vi "Sample Push go for State.vi"(4 "Publish? (T)":bool=TRUE, 6 "Really? (T)":bool=TRUE, 8 "error in (no error)":errorcluster, 9 "State Timeout (Inf=no timeout )":dbl=inf, 10 "Sample Push State":T1=enum."Idle", 11 "cRIO-CO2 in":refnum<class "cRIO-CO2.lvclass">) -> (0 "error out":errorcluster, 3 "cRIO-CO2 out":refnum<class "cRIO-CO2.lvclass">)   [LabVIEW 2015, in "cRIO-Carbondioxide.lvlib" / "cRIO-CO2.lvlib" / "cRIO-CO2.lvclass"]
uses:
  cRIO-CO2.lvclass
  Controls/Sample Push State Enumerator.ctl
  cRIO-CO2.lvclass/cRIO-CO2.ctl
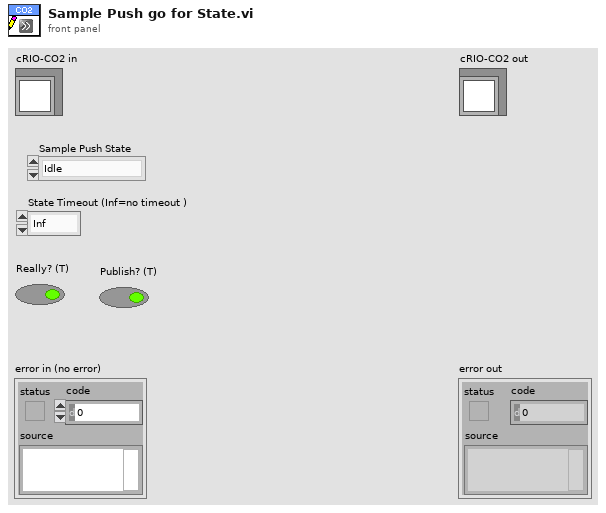
[diagram p1: front panel]
types:
  T1 = typedef "Sample Push State Enumerator.ctl" = enum16{"Undefined", "Initialize", "Dilute", "Close Transfer Line", "Start Heaters", "Warm Up Syringe", "Ready to Push", "Push", "Initiate Stash", "Stash", "Complete", "Abort", "Idle", "Error"}
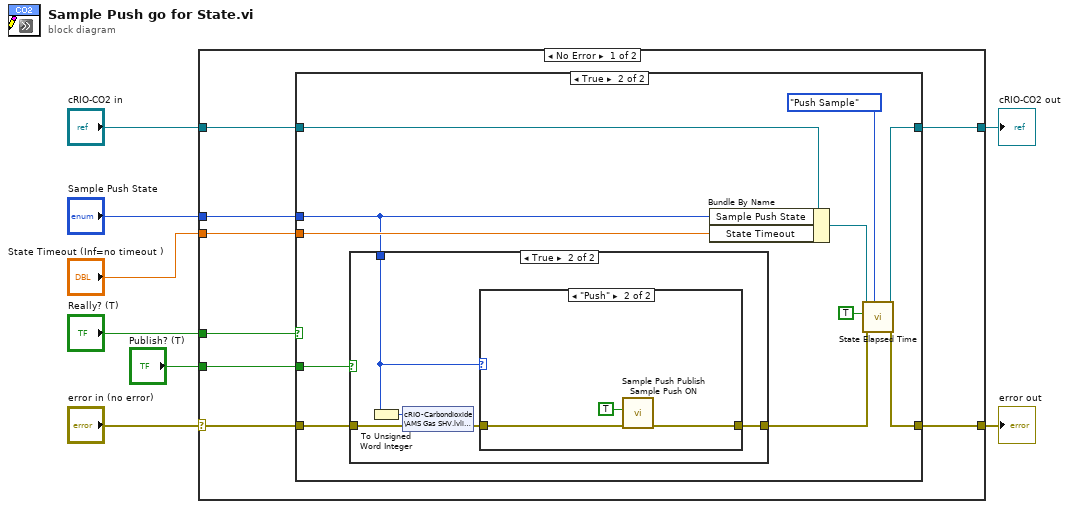
[diagram p0: block diagram]
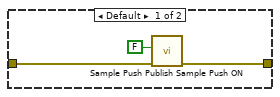
[diagram p4: hidden frame]
diagram:
  n1 = case shown="No Error" "error in (no error)" {
    selector: "error in (no error)" -> [w16 w42]
    tunnel: [w12 w42] -> w7
    tunnel: [w11 w43] -> w5
    tunnel: "cRIO-CO2 in" -> [w14 w43]
    tunnel: "Sample Push State" -> [w15 _]
    tunnel: "State Timeout (Inf=no timeout )" -> [w13 _]
    tunnel: "Really? (T)" -> [w10 _]
    tunnel: "Publish? (T)" -> [w9 _]
    frame No Error {
      n2 = case shown="True" w10 {
        tunnel: w16 -> [w18 w26]
        tunnel: w15 -> [_ w27]
        tunnel: w14 -> [w17 w22]
        tunnel: w13 -> [_ w29]
        tunnel: [w18 w25] -> w12
        tunnel: [w17 w24] -> w11
        tunnel: w9 -> [_ w23]
        frame False {
        }
        frame True {
          n3 = case shown="True" w23 {
            tunnel: w26 -> [w30 w34]
            tunnel: w27 -> [_ w31]
            tunnel: [w30 w32] -> w21
            frame False {
            }
            frame True {
              n4 = To Unsigned Word Integer(number=w31) -> (unsigned 16bit integer=w35:u16)
              n5 = shared-variable "cRIO-Carbondioxide\\AMS Gas SHV.lvlib\\Sample Push.lvlib\\State"(w35, error in=w34) -> (error out=w33:errorcluster)
              n6 = case shown="\"Push\"" w31 {
                tunnel: w33 -> [w38 w41]
                tunnel: [w37 w40] -> w32
                frame Default {
                  n7 = call "Sample Push Publish Sample Push ON.vi"("error in (no error)"=w38, "Sample Push ON"=FALSE) -> ("error out"=w37:errorcluster)  [unwired: 9 in]
                }
                frame "Push" {
                  n8 = call "Sample Push Publish Sample Push ON.vi"("error in (no error)"=w41, "Sample Push ON"=TRUE) -> ("error out"=w40:errorcluster)  [unwired: 9 in]
                }
              }
            }
          }
          n9 = Bundle By Name(cluster=w22, "Sample Push State"=w27, "State Timeout"=w29) -> (w19:refnum<class "cRIO-CO2.lvclass">)
          n10 = call "State Elapsed Time.vi"("State Machine"=enum16{"Transfer Sample", "Push Sample"}."Push Sample", "error in (no error)"=w21, "Reset (F)"=TRUE, "cRIO-CO2 in"=w19) -> ("error out"=w25:errorcluster, "cRIO-CO2 out"=w24:refnum<class "cRIO-CO2.lvclass">)  [unwired: 4 in, 2 out]
        }
      }
    }
    frame Error {
    }
  }
  "error out" <- w7
  "cRIO-CO2 out" <- w5
